vi "FileCheckWithUsing.vi"(8 "错误输入（无错误）":errorcluster, 11 "路径":path) -> (0 "错误输出":errorcluster, 2 "路径副本":path, 3 "file exist":bool)   [LabVIEW 2011]
doc: "和Labview自带函数相比，可检测文件是否被占用，如果被占用，返回false"
uses:
  Data/FileUsingCheck.dll
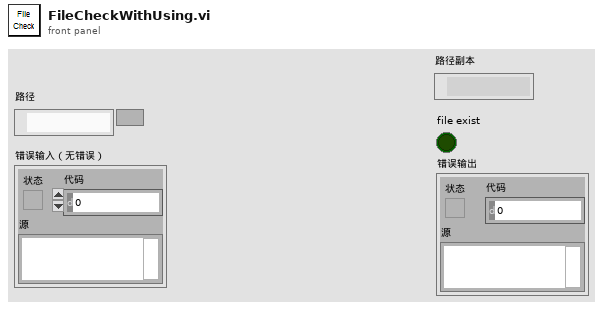
[diagram p1: front panel]
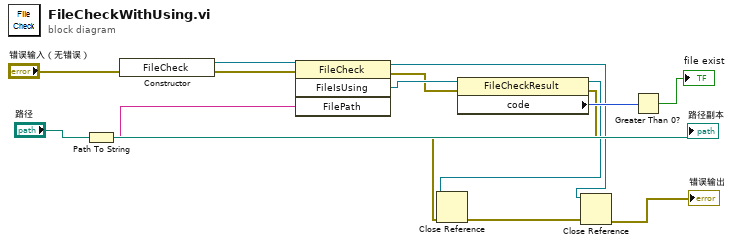
[diagram p0: block diagram]
diagram:
  n1 = Path To String(path="路径") -> (string=w10:string)
  n2 = constructor class="FileCheck"(error in="错误输入（无错误）") -> (reference out=w14:refnum<k24>, error out=w13:errorcluster)  [unwired: 2 in, 1 out]
  n3 = invoke class="FileCheck" method="FileIsUsing"(reference=w14, error in=w13, "FilePath"=w10) -> (reference out=w2:refnum<k24>, error out=w8:errorcluster, "FileIsUsing"=w9:refnum<k24>)  [unwired: 1 in, 1 out]
  n4 = property class="FileCheckResult"(reference=w9, error in=w8) -> (reference out=w4:refnum<k24>, error out=w5:errorcluster, "code"=w7:i32)
  n5 = Close Reference(reference=w4, error in (no error)=w5) -> (error out=w3:errorcluster)
  n6 = Close Reference(reference=w2, error in (no error)=w3) -> (error out=→"错误输出":errorcluster)
  n7 = Greater Than 0?(x=w7) -> (x > 0?=→"file exist":bool)
  "路径副本" <- "路径"
